vi "Defender Goto kick.vi"(6 "d":dbl=110.0, 7 "min dist to kick":dbl=150.0 format="%#_13g", 9 "Bola":dbl[](array[numeric]), 10 "Field Size in":T3, 11 "Our Robot in":T1) -> (3 "Our Robot out":T1)   [LabVIEW 2016]
uses:
  Core/Field Size.ctl
  Core/AI Robot.ctl
  Functions Enum.ctl
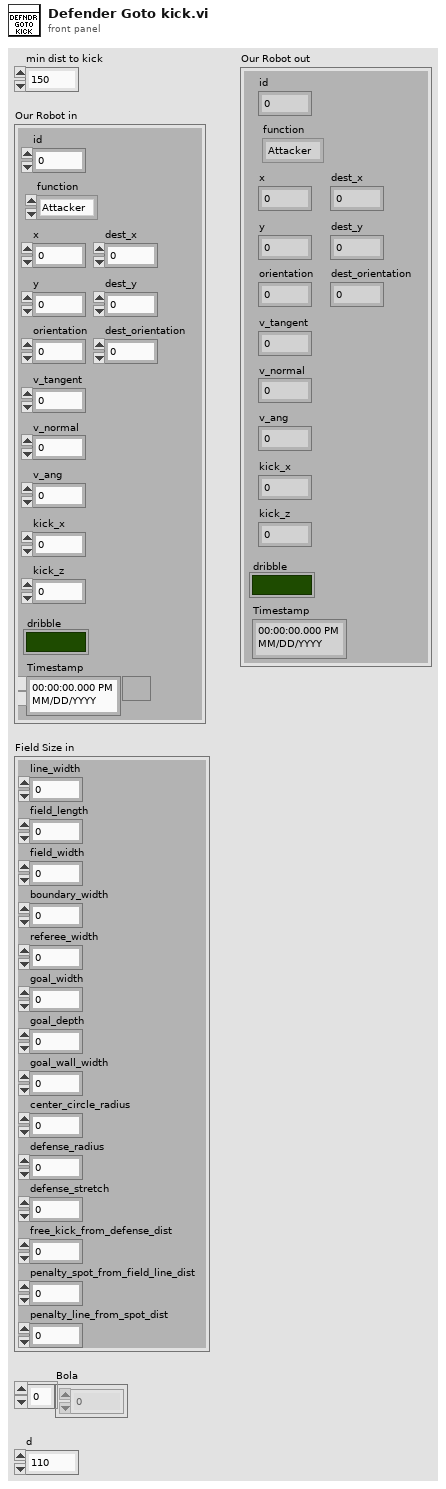
[diagram p1: front panel]
types:
  T1 = typedef "AI Robot.ctl" = cluster{"id":u32, "function":T2, "x":dbl, "y":dbl, "orientation":dbl, "v_tangent":dbl, "v_normal":dbl, "v_ang":dbl, "kick_x":dbl, "kick_z":dbl, "dribble":bool, "Timestamp":timestamp, "dest_x":dbl, "dest_y":dbl, "dest_orientation":dbl}
  T2 = typedef "Functions Enum.ctl" = enum16{"Attacker", "Goalie", "Defender", "Striker", "Goto 0", "Dummy", "ZigZag"}
  T3 = typedef "Field Size.ctl" = cluster{"line_width":u32, "field_length":u32, "field_width":u32, "boundary_width":u32, "referee_width":u32, "goal_width":u32, "goal_depth":u32, "goal_wall_width":u32, "center_circle_radius":u32, "defense_radius":u32, "defense_stretch":u32, "free_kick_from_defense_dist":u32, "penalty_spot_from_field_line_dist":u32, "penalty_line_from_spot_dist":u32}
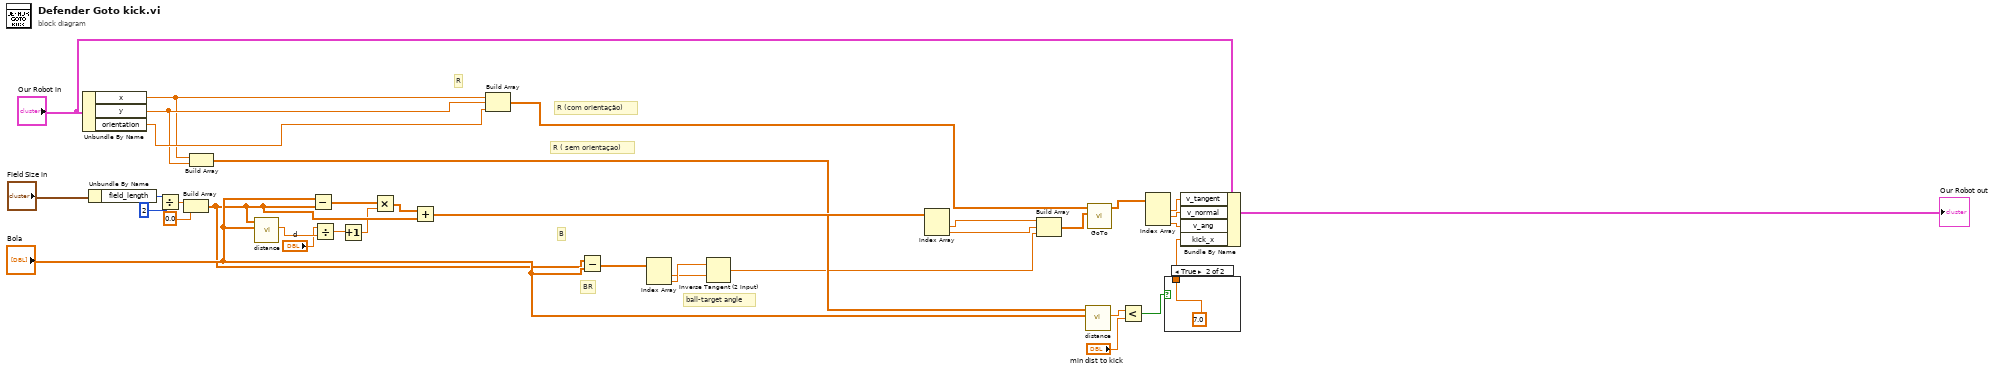
[diagram p0: block diagram]
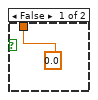
[diagram p2: hidden frame]
diagram:
  # "BR"
  # "ball-target angle"
  # "B"
  # "R ( sem orientaçao)"
  # "R (com orientação)"
  # "R"
  n1 = Unbundle By Name("Our Robot in") -> ("x"=w8:dbl, "y"=w9:dbl, "orientation"=w10:dbl)
  n2 = Unbundle By Name("Field Size in") -> ("field_length"=w6:u32)
  n3 = Divide(x=w6, y=u32 2) -> (x/y=w4:dbl)
  n4 = Build Array(w4, 0.0 ("element")) -> (w35:dbl[])
  n5 = Build Array(w8, w9) -> (w25:dbl[])
  n6 = call "distance.vi"("target pos"="Bola", "obj pos"=w35) -> ("sqrt(x)"=w34:dbl)  [unwired: 9 in]
  n7 = Subtract(x="Bola", y=w35) -> (x-y=w28:dbl[])
  n8 = Divide(x="d", y=w34) -> (x/y=w26:dbl)
  n9 = Increment(x=w26) -> (x+1=w27:dbl)
  n10 = Multiply(x=w28, y=w27) -> (x*y=w29:dbl[])
  n11 = Add(x=w29, y=w35) -> (x+y=w30:dbl[])
  n12 = Build Array(w8, w9, w10) -> (w24:dbl[])
  n13 = Subtract(x=w35, y="Bola") -> (x-y=w17:dbl[])
  n14 = Index Array(array=w17) -> (element #1=w15:dbl, element #2=w16:dbl)  [unwired: 2 in]
  n15 = Inverse Tangent (2 Input)(1:w15, 2:w16) -> (0:w18:dbl)
  n16 = Index Array(array=w30) -> (element #1=w31:dbl, element #2=w32:dbl)  [unwired: 2 in]
  n17 = Build Array(w31, w32, w18) -> (w19:dbl[])
  n18 = call "distance.vi"("target pos"="Bola", "obj pos"=w25) -> ("sqrt(x)"=w11:dbl)  [unwired: 9 in]
  n19 = call "GoTo.vi"("Target"=w19, "Position"=w24) -> ("Output\nVelocity"=w20:dbl[])  [unwired: 8 in, 1 out]
  n20 = Less?(x=w11, y="min dist to kick") -> (x < y?=w13:bool)
  n21 = Index Array(array=w20) -> (element #1=w21:dbl, element #2=w22:dbl, element #3=w23:dbl)  [unwired: 3 in]
  n22 = case shown="True" w13 {
    tunnel: [0.0 7.0] -> w12
    frame False {
    }
    frame True {
    }
  }
  n23 = Bundle By Name(cluster="Our Robot in", "v_tangent"=w21, "v_normal"=w22, "v_ang"=w23, "kick_x"=w12) -> (→"Our Robot out":T1)
